vi "Build NT Dbl Buffer.vi"(11 "Double":dbl) -> (3 "Data Buffer":string)   [LabVIEW 2017]
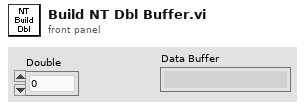
[diagram p1: front panel]
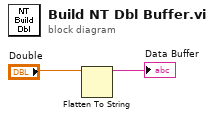
[diagram p0: block diagram]
diagram:
  n1 = Flatten To String(anything="Double") -> (data string=→"Data Buffer":string)  [unwired: 3 in, 2 out]
